vi "Graph ploting data.vi"() -> ()   [LabVIEW 2015]
panel:
  out "XY Graph":cluster{"Y":dbl[], "Y":dbl[]}[](graph)
  # "Graph ploting data"
  # "Pardeep Kumar"
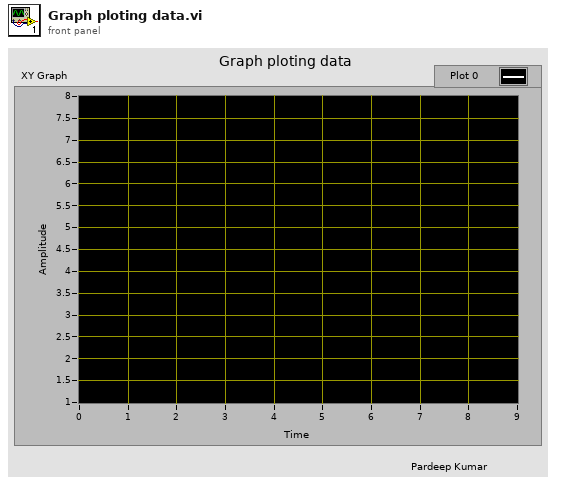
[diagram p1: front panel]
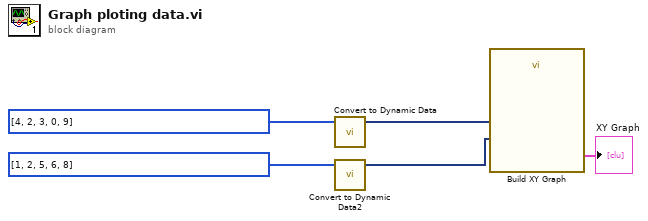
[diagram p0: block diagram]
diagram:
  n1 = call "Convert to Dynamic Data"("Array"=i32[] [4, 2, 3, 0, 9]) -> ("Dynamic Data Type"=w5:dynamicdata)  [unwired: 3 in]
  n2 = call "Convert to Dynamic Data2"("Array"=i32[] [1, 2, 5, 6, 8]) -> ("Dynamic Data Type"=w4:dynamicdata)  [unwired: 3 in]
  n3 = call "Build XY Graph"("Y Input"=w4, "X Input"=w5) -> ("XY Graph"=→"XY Graph":cluster{"Y":dbl[], "Y":dbl[]}[])  [unwired: 3 in, 6 out]
